vi "HEUI_Event_FGV.vi"(0 "Event In":refnum<user-event>, 7 "Action":enum16{"Get", "Set"}(ring), 11 "Error In":errorcluster) -> (4 "Event Out":refnum<user-event>, 15 "Error Out":errorcluster)   [LabVIEW 2023]
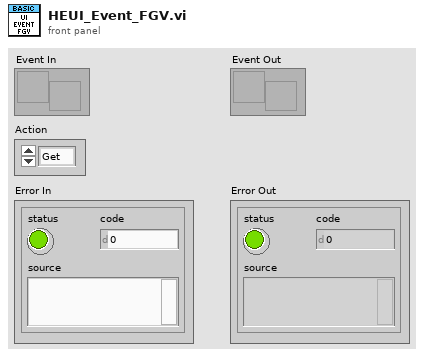
[diagram p1: front panel]
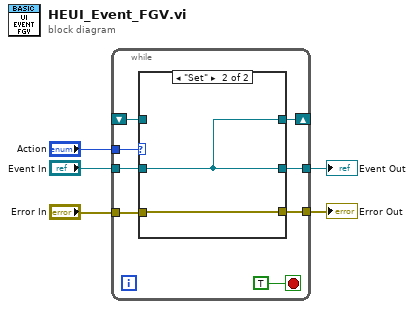
[diagram p0: block diagram]
diagram:
  n1 = while {
    tunnel: "Error In" -> [w12]
    tunnel: [w11] -> w4
    tunnel: "Action" -> [w10]
    shift-right: [w6] -> _
    shift-left: _ -> [w7]
    tunnel: "Event In" -> [w9]
    tunnel: [w8] -> w1
    stop <- TRUE stop-if-true
    n2 = case shown="\"Set\"" w10 {
      tunnel: w12 -> [w15 w17]
      tunnel: [w15 w17] -> w11
      tunnel: w9 -> [_ w16]
      tunnel: [w14 w16] -> w8
      tunnel: w7 -> [w14 _]
      tunnel: [w14 w16] -> w6
      frame "Get", Default {
      }
      frame "Set" {
      }
    }
  }
  "Error Out" <- w4
  "Event Out" <- w1
